vi "OldClient.vi"() -> ()   [LabVIEW 2025]
uses:
  common/CommonClientNetworkInterfaceGlobalVariables.vi
  ClientGlobalVariables.vi
  ClientNetworkInterfaceGlobalVariables.vi
panel:
  out "ACTION":T1
  in  "Array":string[][](array[string])
  in  "Team":u8=1 max=15 step=1
  in  "Tab Control":enum32{"start", "PreGame", "InGame"}(tab)
  in  "ServerAddress":string
  in  "exit":bool
  in  "play":bool
  out "Status":string
  in  "PlayerName":string
  in  "leave game":bool
  in  "PreGame menu":enum32{"Team", "Options"}(tab)
  in  "spectator":bool caption="Blank Button"
  in  "team5":bool caption="Blank Button"
  in  "team4":bool caption="Blank Button"
  in  "team3":bool caption="Blank Button"
  in  "team2":bool caption="Blank Button"
  in  "team1":bool caption="Blank Button"
  out "Lobby Player List":T2(array[cluster])
  in  "Speed":i32(slide) caption="Slide" scale=1.0..4.0
  in  "Map Width":i32(slide) caption="Slide" scale=10.0..40.0
  in  "Map Height":i32(slide) caption="Slide" scale=10.0..40.0
  in  "City Density":i32(slide) caption="Slide" scale=20.0..80.0
  in  "Mountain Density":i32(slide) caption="Slide" scale=20.0..80.0
  out "Status 2":string
  in  "Ready":bool
  in  "back_to _lobby":bool
  out "Turns":string
  in  "play 2":bool
  out "Game Field":picture
  out "In-game Player List":string[][](table) caption="Table Control"
  # "generals.io"
  # "generals.io"
  # "Protect your general. Capture enemy generals."
  # "Player Name"
  # "Server Address"
  # "Status"
  # "Status"
  # "select your team"
  # "Team"
  # "Turn"
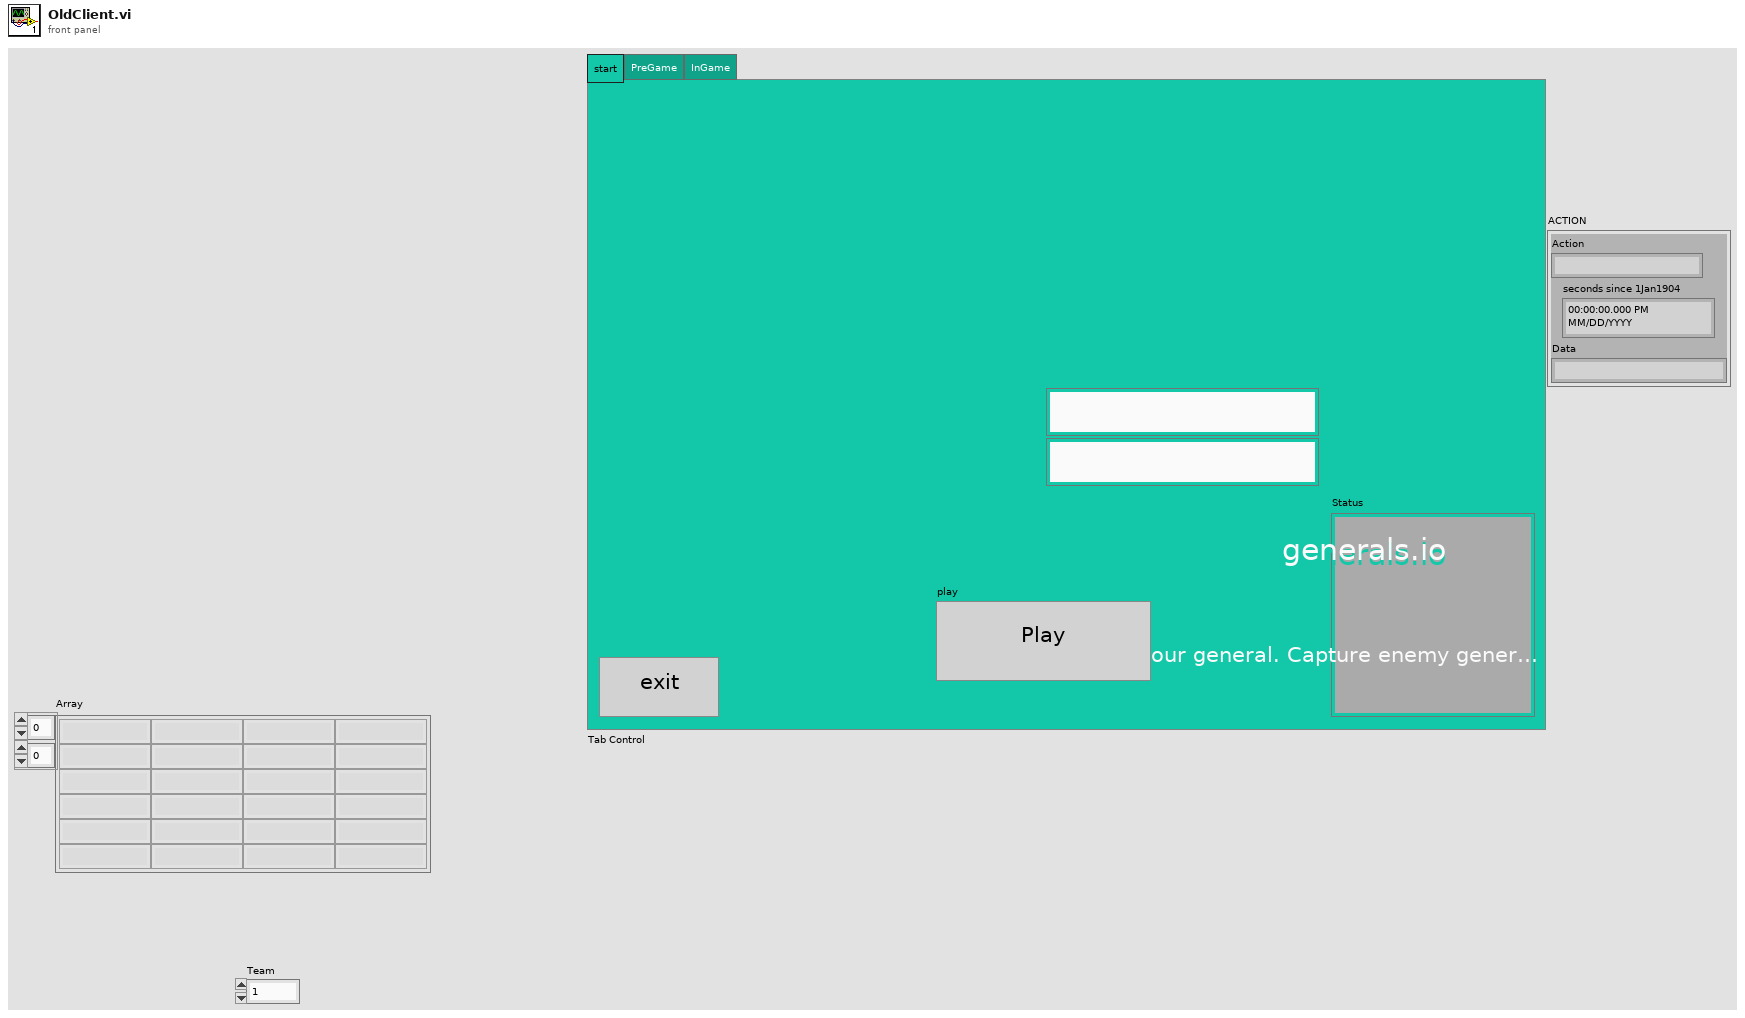
[diagram p1: front panel]
types:
  T1 = cluster{"Action":string, "seconds since 1Jan1904":timestamp, "Data":string}
  T2 = cluster{"Color":u32, "Host":bool, "Name":string, "Team":u8, "Ready":bool}[]
  T3 = cluster{"seconds since 1Jan1904":timestamp, "Data":string}
  T4 = enum16{"Wait Send Queue Ready", "Wait Receive Queue Ready", "Poll Read Queue", "Process Data"}
  T5 = typedef "LVPoint32TypeDef.ctl" = cluster{"Horizontal":i32, "Vertical":i32}
  T6 = cluster{"Round":u32, "FieldArray":cluster{"Troops":u32, "Owner":i32, "Mountain":bool, "City":bool, "General":bool, "Fog":bool}[][]}
  T7 = cluster{"Troops":u32, "Owner":i32, "Mountain":bool, "City":bool, "General":bool, "Fog":bool}[][]
  T8 = map{u32, cluster{"Name":string, "Team":u8, "Ready":bool, "Host":bool, "Alive":bool, "Color":u32, "Lands":set{cluster{"Row":u32, "Column":u32}}, "Army":u32}}
  T9 = cluster{"Color":u32, "Host":bool, "Name":string, "Team":u8, "Ready":bool}
  T10 = cluster{"Lands":set{cluster{"Row":u32, "Column":u32}}}[]
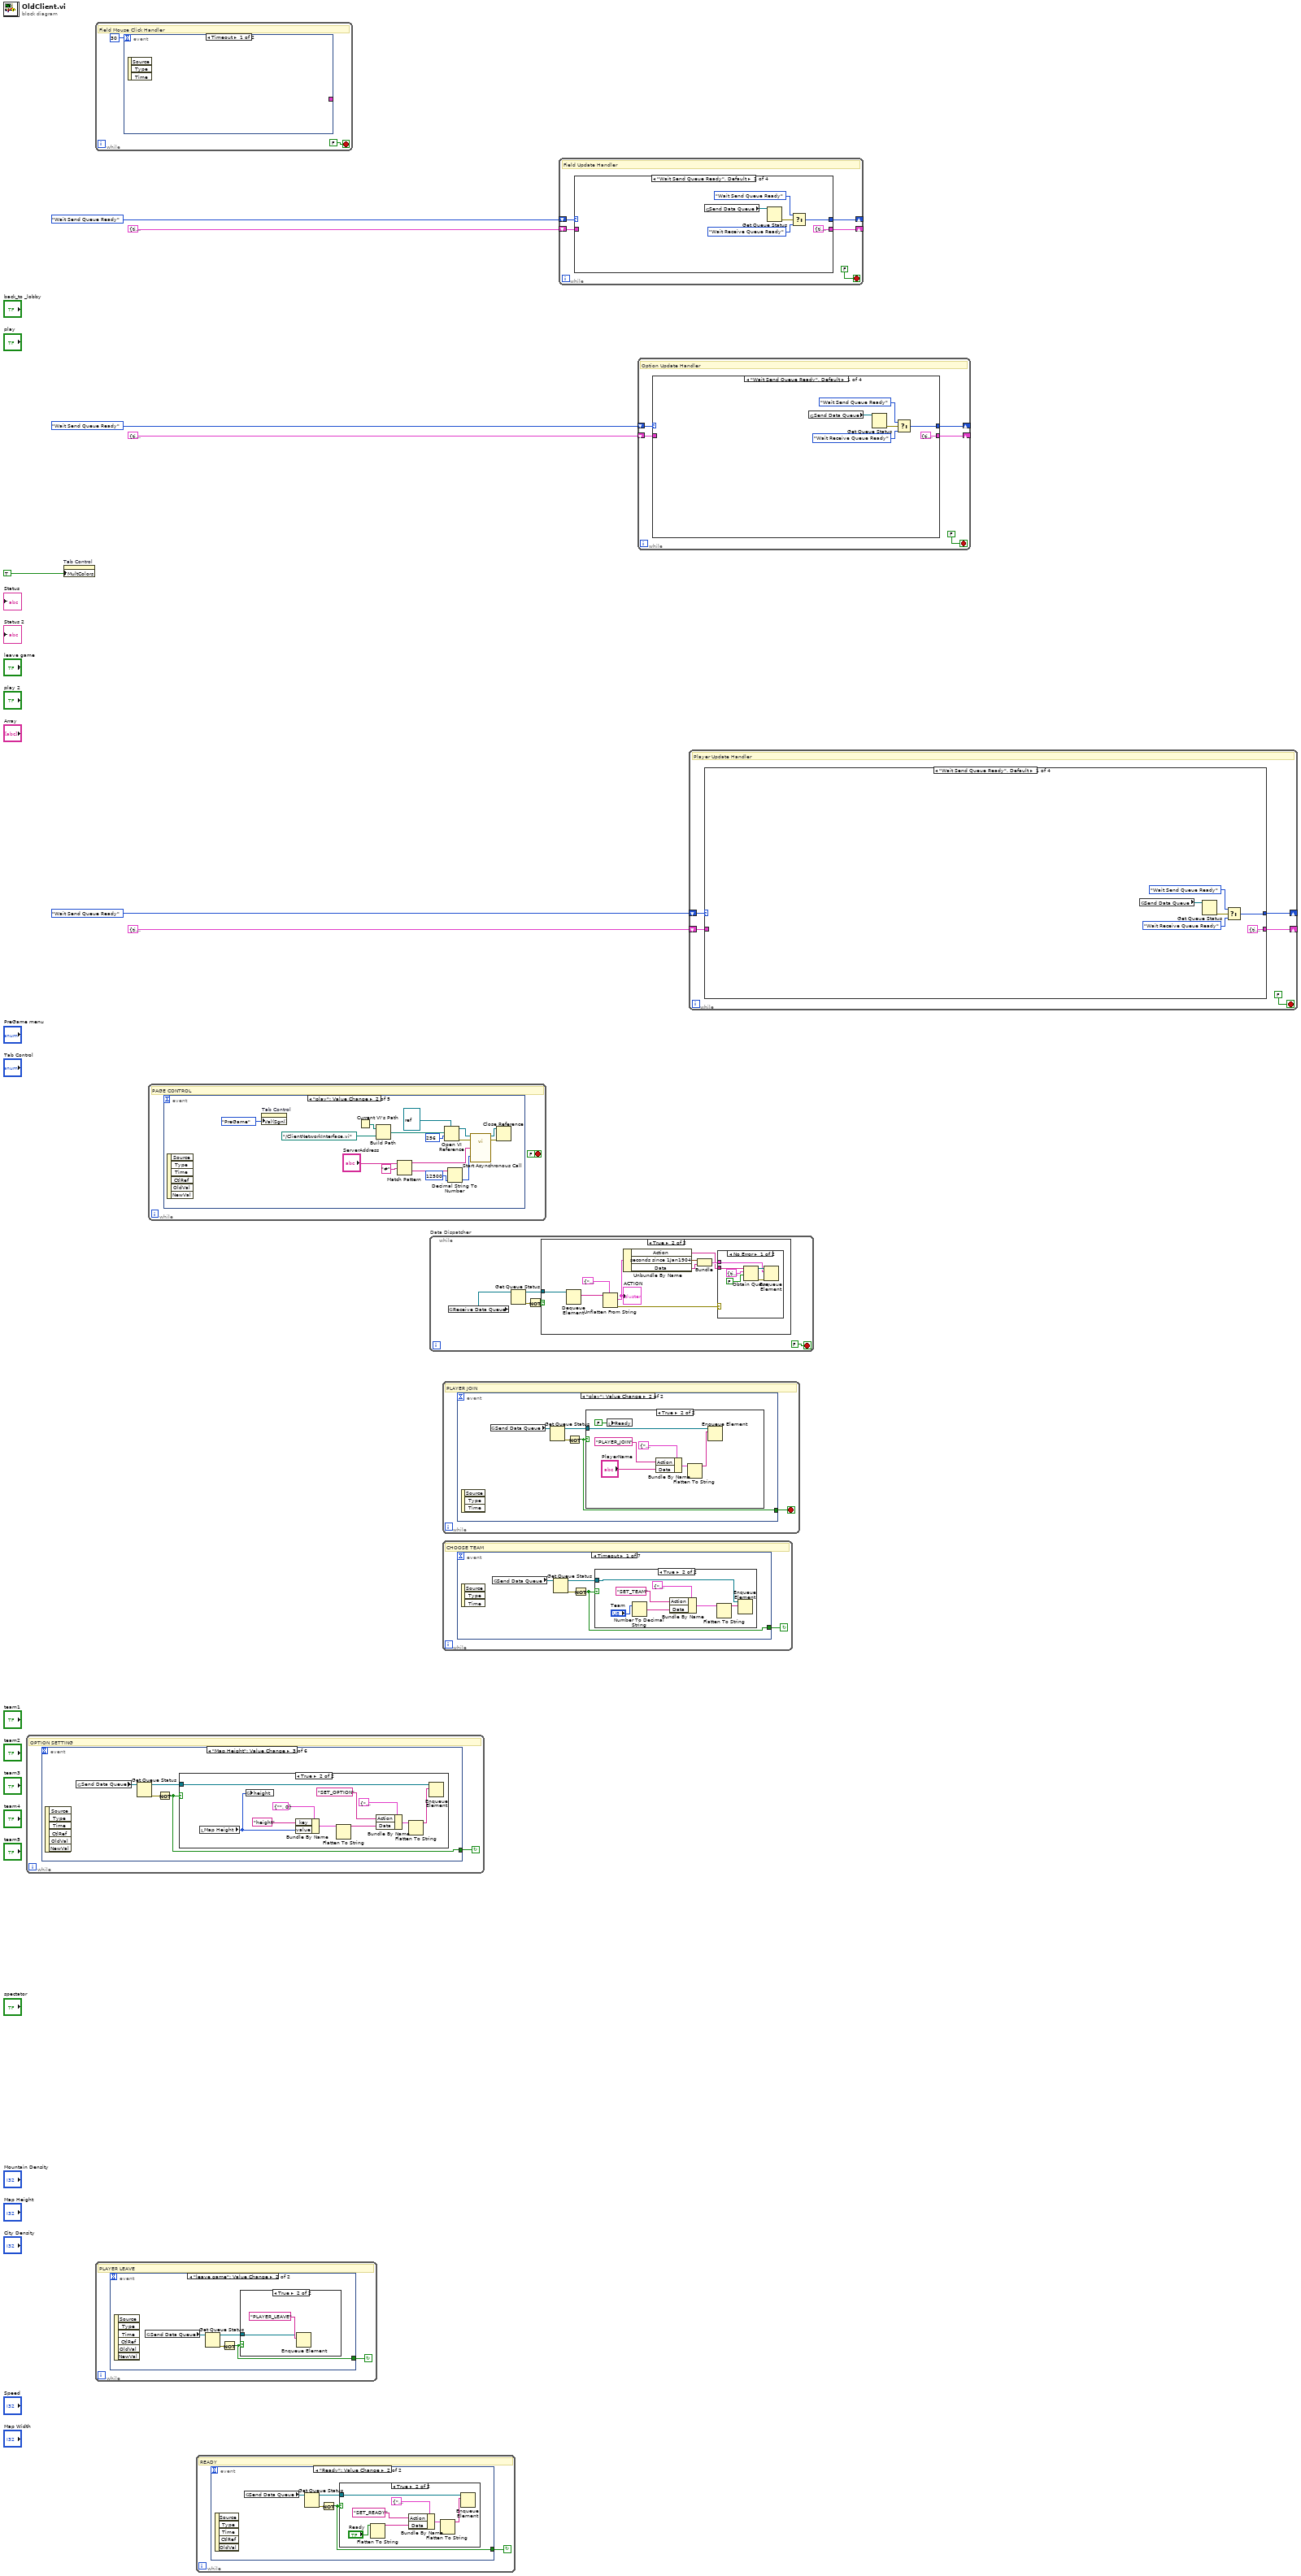
[diagram p0: block diagram]
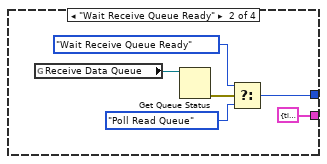
[diagram p2: hidden frame]
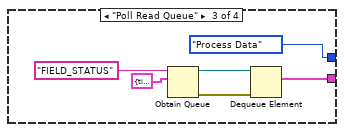
[diagram p3: hidden frame]
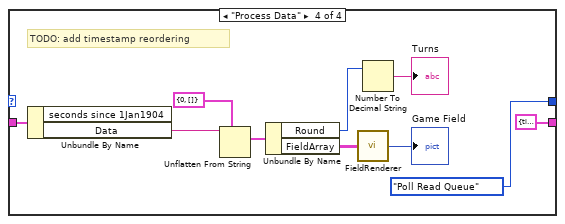
[diagram p4: hidden frame]
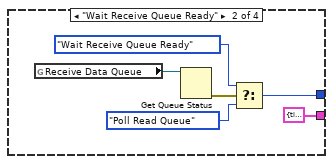
[diagram p5: hidden frame]
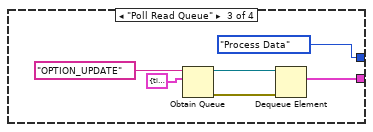
[diagram p6: hidden frame]
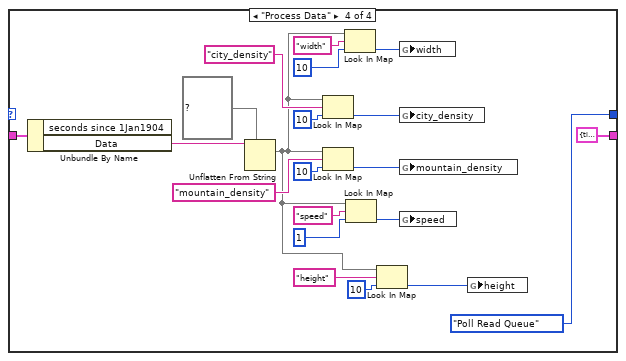
[diagram p7: hidden frame]
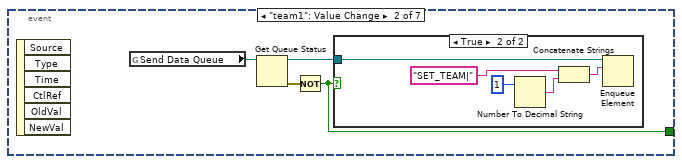
[diagram p9: hidden frame]
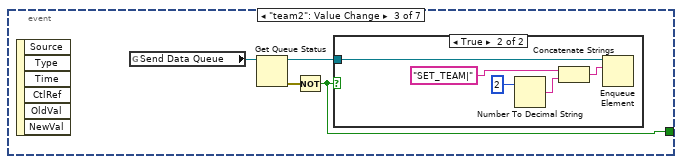
[diagram p11: hidden frame]
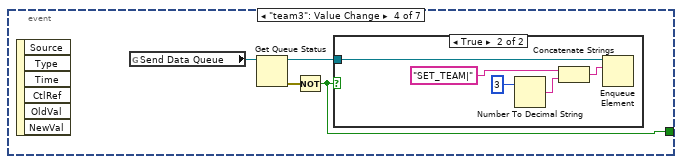
[diagram p13: hidden frame]
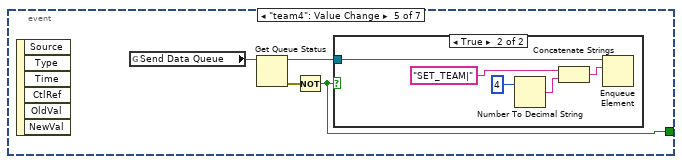
[diagram p15: hidden frame]
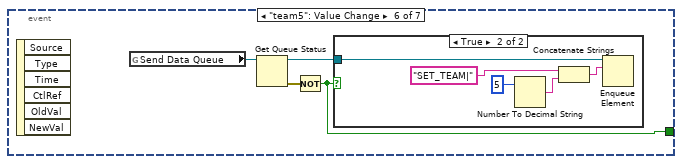
[diagram p17: hidden frame]
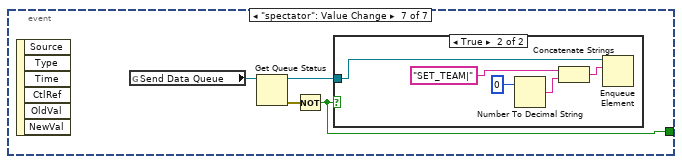
[diagram p19: hidden frame]
diagram:
  n1 = while {
    stop <- w8 continue-if-true
    # "OPTION SETTING"
    n2 = event shown="[2] \"Map Height\": Value Change" {
      selector: _ -> [_ _ _ _ _ _]
      dyn-events: _ -> [_ _ _ _ _ _]
      timeout: _ -> [_ _ _ _ _ _]
      tunnel: [_ w9 w24 w37 w51 w66] -> w8
      event Timeout {
        n3 = event-data() -> ()  [unwired: 1 in, 3 out]
      }
      event "Map Width": Value Change {
        n4 = event-data() -> ()  [unwired: 1 in, 6 out]
        n5 = global read "CommonClientNetworkInterfaceGlobalVariables.vi" "Send Data Queue"() -> (w11:refnum<queue>)
        n6 = Get Queue Status(queue=w11) -> (queue out=w10:refnum<queue>, error out=w12:errorcluster)  [unwired: 2 in, 6 out]
        n7 = Not(x=w12) -> (.not. x?=w9:bool)
        n8 = case shown="True" w9 {
          tunnel: w10 -> [_ w22]
          frame False {
          }
          frame True {
            n9 = local read "Map Width"() -> (w19:i32)
            n10 = global write "ClientGlobalVariables.vi" "width"(w19) -> ()
            n11 = Bundle By Name(cluster=cluster{"key":string, "value":u32} {"key"="", "value"=0}, "key"="width" ("Option"), "value"=w19) -> (w15:cluster{"key":string, "value":u32})
            n12 = Flatten To String(anything=w15) -> (data string=w16:string)  [unwired: 3 in, 2 out]
            n13 = Bundle By Name(cluster=cluster{"Action":string, "Data":string} {"Action"="", "Data"=""} ("CommandCluster"), "Action"="SET_OPTION" ("string"), "Data"=w16) -> (w13:cluster{"Action":string, "Data":string})
            n14 = Flatten To String(anything=w13) -> (data string=w14:string)  [unwired: 3 in, 2 out]
            n15 = Enqueue Element(queue=w22, element=w14) -> ()  [unwired: 2 in, 3 out]
          }
        }
      }
      event "Map Height": Value Change {
        n16 = event-data() -> ()  [unwired: 1 in, 6 out]
        n17 = global read "CommonClientNetworkInterfaceGlobalVariables.vi" "Send Data Queue"() -> (w25:refnum<queue>)
        n18 = Get Queue Status(queue=w25) -> (queue out=w23:refnum<queue>, error out=w26:errorcluster)  [unwired: 2 in, 6 out]
        n19 = Not(x=w26) -> (.not. x?=w24:bool)
        n20 = case shown="True" w24 {
          tunnel: w23 -> [_ w28]
          frame False {
          }
          frame True {
            n21 = local read "Map Height"() -> (w27:i32)
            n22 = global write "ClientGlobalVariables.vi" "height"(w27) -> ()
            n23 = Bundle By Name(cluster=cluster{"key":string, "value":u32} {"key"="", "value"=0}, "key"="height" ("Option"), "value"=w27) -> (w31:cluster{"key":string, "value":u32})
            n24 = Flatten To String(anything=w31) -> (data string=w32:string)  [unwired: 3 in, 2 out]
            n25 = Bundle By Name(cluster=cluster{"Action":string, "Data":string} {"Action"="", "Data"=""} ("CommandCluster"), "Action"="SET_OPTION" ("string"), "Data"=w32) -> (w29:cluster{"Action":string, "Data":string})
            n26 = Flatten To String(anything=w29) -> (data string=w30:string)  [unwired: 3 in, 2 out]
            n27 = Enqueue Element(queue=w28, element=w30) -> ()  [unwired: 2 in, 3 out]
          }
        }
      }
      event "Speed": Value Change {
        n28 = event-data() -> ()  [unwired: 1 in, 6 out]
        n29 = global read "CommonClientNetworkInterfaceGlobalVariables.vi" "Send Data Queue"() -> (w39:refnum<queue>)
        n30 = Get Queue Status(queue=w39) -> (queue out=w38:refnum<queue>, error out=w40:errorcluster)  [unwired: 2 in, 6 out]
        n31 = Not(x=w40) -> (.not. x?=w37:bool)
        n32 = case shown="True" w37 {
          tunnel: w38 -> [_ w41]
          frame False {
          }
          frame True {
            n33 = local read "Speed"() -> (w42:i32)
            n34 = global write "ClientGlobalVariables.vi" "speed"(w42) -> ()
            n35 = Bundle By Name(cluster=cluster{"key":string, "value":u32} {"key"="", "value"=0}, "key"="speed" ("Option"), "value"=w42) -> (w45:cluster{"key":string, "value":u32})
            n36 = Flatten To String(anything=w45) -> (data string=w46:string)  [unwired: 3 in, 2 out]
            n37 = Bundle By Name(cluster=cluster{"Action":string, "Data":string} {"Action"="", "Data"=""} ("CommandCluster"), "Action"="SET_OPTION" ("string"), "Data"=w46) -> (w43:cluster{"Action":string, "Data":string})
            n38 = Flatten To String(anything=w43) -> (data string=w44:string)  [unwired: 3 in, 2 out]
            n39 = Enqueue Element(queue=w41, element=w44) -> ()  [unwired: 2 in, 3 out]
          }
        }
      }
      event "Mountain Density": Value Change {
        n40 = event-data() -> ()  [unwired: 1 in, 6 out]
        n41 = global read "CommonClientNetworkInterfaceGlobalVariables.vi" "Send Data Queue"() -> (w53:refnum<queue>)
        n42 = Get Queue Status(queue=w53) -> (queue out=w52:refnum<queue>, error out=w54:errorcluster)  [unwired: 2 in, 6 out]
        n43 = Not(x=w54) -> (.not. x?=w51:bool)
        n44 = case shown="True" w51 {
          tunnel: w52 -> [_ w56]
          frame False {
          }
          frame True {
            n45 = local read "Mountain Density"() -> (w55:i32)
            n46 = global write "ClientGlobalVariables.vi" "mountain_density"(w55) -> ()
            n47 = Bundle By Name(cluster=cluster{"key":string, "value":u32} {"key"="", "value"=0}, "key"="mountain_density" ("Option"), "value"=w55) -> (w59:cluster{"key":string, "value":u32})
            n48 = Flatten To String(anything=w59) -> (data string=w60:string)  [unwired: 3 in, 2 out]
            n49 = Bundle By Name(cluster=cluster{"Action":string, "Data":string} {"Action"="", "Data"=""} ("CommandCluster"), "Action"="SET_OPTION" ("string"), "Data"=w60) -> (w57:cluster{"Action":string, "Data":string})
            n50 = Flatten To String(anything=w57) -> (data string=w58:string)  [unwired: 3 in, 2 out]
            n51 = Enqueue Element(queue=w56, element=w58) -> ()  [unwired: 2 in, 3 out]
          }
        }
      }
      event "City Density": Value Change {
        n52 = event-data() -> ()  [unwired: 1 in, 6 out]
        n53 = global read "CommonClientNetworkInterfaceGlobalVariables.vi" "Send Data Queue"() -> (w67:refnum<queue>)
        n54 = Get Queue Status(queue=w67) -> (queue out=w65:refnum<queue>, error out=w68:errorcluster)  [unwired: 2 in, 6 out]
        n55 = Not(x=w68) -> (.not. x?=w66:bool)
        n56 = case shown="True" w66 {
          tunnel: w65 -> [_ w69]
          frame False {
          }
          frame True {
            n57 = local read "City Density"() -> (w70:i32)
            n58 = global write "ClientGlobalVariables.vi" "city_density"(w70) -> ()
            n59 = Bundle By Name(cluster=cluster{"key":string, "value":u32} {"key"="", "value"=0}, "key"="city_density" ("Option"), "value"=w70) -> (w73:cluster{"key":string, "value":u32})
            n60 = Flatten To String(anything=w73) -> (data string=w74:string)  [unwired: 3 in, 2 out]
            n61 = Bundle By Name(cluster=cluster{"Action":string, "Data":string} {"Action"="", "Data"=""} ("CommandCluster"), "Action"="SET_OPTION" ("string"), "Data"=w74) -> (w71:cluster{"Action":string, "Data":string})
            n62 = Flatten To String(anything=w71) -> (data string=w72:string)  [unwired: 3 in, 2 out]
            n63 = Enqueue Element(queue=w69, element=w72) -> ()  [unwired: 2 in, 3 out]
          }
        }
      }
    }
  }
  n64 = property on="Tab Control" class="TabCtl (strict)"("MultColors"=TRUE ("Allow Multiple Colors")) -> ()  [unwired: 2 in, 2 out]
  n65 = while {
    stop <- FALSE stop-if-true
    # "Field Mouse Click Handler"
    n66 = event shown="[0] Timeout" {
      selector: _ -> [_ _]
      dyn-events: _ -> [_ _]
      timeout: 30 -> [_ _]
      tunnel: [_ w94] -> _
      event Timeout {
        n67 = event-data() -> ()  [unwired: 1 in, 3 out]
      }
      event "Game Field": Mouse Down {
        # "col"
        # "row"
        n68 = event-data() -> ("Coords"=w96:T5)  [unwired: 1 in, 7 out]
        n69 = Unbundle By Name(w96) -> ("Horizontal"=w93:i32, "Vertical"=w92:i32)
        n70 = global read "ClientGlobalVariables.vi" "FieldLength"() -> (w83:i32)
        n71 = global read "ClientGlobalVariables.vi" "height"() -> (w84:i32)
        n72 = global read "ClientGlobalVariables.vi" "width"() -> (w85:i32)
        n73 = Quotient & Remainder(x=w83, y=w85) -> (floor(x/y)=w82:i32)  [unwired: 1 out]
        n74 = Quotient & Remainder(x=w83, y=w84) -> (floor(x/y)=w81:i32)  [unwired: 1 out]
        n75 = Quotient & Remainder(x=w93, y=w82) -> (floor(x/y)=w90:i32)  [unwired: 1 out]
        n76 = Quotient & Remainder(x=w92, y=w81) -> (floor(x/y)=w88:i32)  [unwired: 1 out]
        n77 = Subtract(x=w88, y=4) -> (x-y=w87:i32)
        n78 = Subtract(x=w90, y=13) -> (x-y=w91:i32)
        n79 = Bundle(w91, w87, TRUE) -> (w94:cluster{i32, i32, bool})  [unwired: 1 in]
      }
    }
  }
  n80 = while {
    stop <- w97 continue-if-true
    # "PLAYER LEAVE"
    n81 = event shown="[1] \"leave game\": Value Change" {
      selector: _ -> [_ _]
      dyn-events: _ -> [_ _]
      timeout: _ -> [_ _]
      tunnel: [_ w99] -> w97
      event Timeout {
        n82 = event-data() -> ()  [unwired: 1 in, 3 out]
      }
      event "leave game": Value Change {
        n83 = event-data() -> ()  [unwired: 1 in, 6 out]
        n84 = global read "CommonClientNetworkInterfaceGlobalVariables.vi" "Send Data Queue"() -> (w100:refnum<queue>)
        n85 = Get Queue Status(queue=w100) -> (queue out=w98:refnum<queue>, error out=w101:errorcluster)  [unwired: 2 in, 6 out]
        n86 = Not(x=w101) -> (.not. x?=w99:bool)
        n87 = case shown="True" w99 {
          tunnel: w98 -> [_ w102]
          frame False {
          }
          frame True {
            n88 = Enqueue Element(queue=w102, element="PLAYER_LEAVE" ("string")) -> ()  [unwired: 2 in, 3 out]
          }
        }
      }
    }
  }
  n89 = while {
    stop <- FALSE stop-if-true
    # "PAGE CONTROL"
    n90 = event shown="[1] \"play\": Value Change" {
      selector: _ -> [_ _ _ _ _]
      dyn-events: _ -> [_ _ _ _ _]
      timeout: _ -> [_ _ _ _ _]
      event Timeout {
        n91 = event-data() -> ()  [unwired: 1 in, 3 out]
      }
      event "play": Value Change {
        n92 = event-data() -> ()  [unwired: 1 in, 6 out]
        n93 = property on="Tab Control" class="TabCtl (strict)"("Val(Sgnl)"=enum32{"start", "PreGame", "InGame"}."PreGame" ("Value (Signaling)")) -> ()  [unwired: 2 in, 2 out]
        n94 = Current VI's Path() -> (path=w115:path)
        n95 = Build Path(base path=w115, name or relative path=path "../ClientNetworkInterface.vi" ("vi path")) -> (appended path=w113:path)
        n96 = Match Pattern(string="ServerAddress", regular expression="#") -> (before substring=w106:string, after substring=w119:string)  [unwired: 1 in, 2 out]
        n97 = Open VI Reference(type specifier VI Refnum (for type only)=refnum<vi> refnum ("VI Refnum"), vi path=w113, options=256) -> (vi reference=w107:refnum<vi>, error out=w111:errorcluster)  [unwired: 3 in]
        n98 = Decimal String To Number(string=w119, default (0L)=u16 12500 ("Server Port")) -> (number=w105:u16)  [unwired: 1 in, 1 out]
        n99 = call-by-ref "Start Asynchronous Call"(reference=w107, error in=w111, "Server Port"=w105, "Server Address"=w106) -> (reference out=w110:refnum<vi>, error out=w109:errorcluster)
        n100 = Close Reference(reference=w110, error in (no error)=w109) -> ()  [unwired: 1 out]
      }
      event "leave game": Value Change {
        n101 = event-data() -> ()  [unwired: 1 in, 6 out]
        n102 = property on="Tab Control" class="TabCtl (strict)"("Val(Sgnl)"=enum32{"start", "PreGame", "InGame"}."start" ("Value (Signaling)")) -> ()  [unwired: 2 in, 2 out]
      }
      event "back_to _lobby": Value Change {
        n103 = event-data() -> ()  [unwired: 1 in, 6 out]
        n104 = local read "Speed"() -> (w126:i32)
        n105 = local read "Map Height"() -> (w125:i32)
        n106 = local read "City Density"() -> (w123:i32)
        n107 = local read "Map Width"() -> (w124:i32)
        n108 = global write "ClientGlobalVariables.vi" "FieldLength"(600 ("FieldLength")) -> ()
        n109 = global write "ClientGlobalVariables.vi" "speed"(w126) -> ()
        n110 = local read "Mountain Density"() -> (w127:i32)
        n111 = global write "ClientGlobalVariables.vi" "city_density"(w123) -> ()
        n112 = global write "ClientGlobalVariables.vi" "height"(w125) -> ()
        n113 = global write "ClientGlobalVariables.vi" "width"(w124) -> ()
        n114 = property on="Tab Control" class="TabCtl (strict)"("Val(Sgnl)"=enum32{"start", "PreGame", "InGame"}."PreGame" ("Value (Signaling)")) -> ()  [unwired: 2 in, 2 out]
        n115 = global write "ClientGlobalVariables.vi" "mountain_density"(w127) -> ()
      }
      event "exit": Value Change {
        n116 = event-data() -> ()  [unwired: 1 in, 6 out]
        n117 = Quit LabVIEW(quit? (T)="exit") -> ()
      }
    }
  }
  n118 = while {
    stop <- w130 continue-if-true
    # "READY"
    n119 = event shown="[1] \"Ready\": Value Change" {
      selector: _ -> [_ _]
      dyn-events: _ -> [_ _]
      timeout: _ -> [_ _]
      tunnel: [_ w131] -> w130
      event Timeout {
        n120 = event-data() -> ()  [unwired: 1 in, 3 out]
      }
      event "Ready": Value Change {
        n121 = event-data() -> ()  [unwired: 1 in, 5 out]
        n122 = global read "CommonClientNetworkInterfaceGlobalVariables.vi" "Send Data Queue"() -> (w134:refnum<queue>)
        n123 = Get Queue Status(queue=w134) -> (queue out=w133:refnum<queue>, error out=w132:errorcluster)  [unwired: 2 in, 6 out]
        n124 = Not(x=w132) -> (.not. x?=w131:bool)
        n125 = case shown="True" w131 {
          tunnel: w133 -> [_ w135]
          frame False {
          }
          frame True {
            n126 = Flatten To String(anything="Ready") -> (data string=w139:string)  [unwired: 3 in, 2 out]
            n127 = Bundle By Name(cluster=cluster{"Action":string, "Data":string} {"Action"="", "Data"=""} ("CommandCluster"), "Action"="SET_READY" ("string"), "Data"=w139) -> (w137:cluster{"Action":string, "Data":string})
            n128 = Flatten To String(anything=w137) -> (data string=w138:string)  [unwired: 3 in, 2 out]
            n129 = Enqueue Element(queue=w135, element=w138) -> ()  [unwired: 2 in, 3 out]
          }
        }
      }
    }
  }
  n130 = while "Data Dispatcher" {
    stop <- FALSE stop-if-true
    n131 = global read "ClientNetworkInterfaceGlobalVariables.vi" "Receive Data Queue"() -> (w142:refnum<queue>)
    n132 = Get Queue Status(queue=w142) -> (queue out=w143:refnum<queue>, error out=w145:errorcluster)  [unwired: 2 in, 6 out]
    n133 = Not(x=w145) -> (.not. x?=w144:bool)
    n134 = case shown="True" w144 {
      tunnel: w143 -> [_ w155]
      frame False {
      }
      frame True {
        n135 = Dequeue Element(queue=w155) -> (element=w154:string)  [unwired: 2 in, 3 out]
        n136 = Unflatten From String(type=T1 {"Action"="", "seconds since 1Jan1904"=timestamp(0 s since 1904-01-01), "Data"=""} ("CommandCluster"), binary string=w154) -> (value=w147:T1, error out=w148:errorcluster)  [unwired: 3 in, 1 out]
        "ACTION" <- w147
        n137 = Unbundle By Name(w147) -> ("Action"=w149:string, "seconds since 1Jan1904"=w152:timestamp, "Data"=w151:string)
        n138 = Bundle("seconds since 1Jan1904"=w152, "Data"=w151) -> (w150:T3)  [unwired: 1 in]
        n139 = case shown="No Error" w148 {
          tunnel: w150 -> [w158 _]
          tunnel: w149 -> [w157 _]
          frame No Error {
            n140 = Obtain Queue(name (unnamed)=w157, element data type=T3 {"seconds since 1Jan1904"=timestamp(0 s since 1904-01-01), "Data"=""} ("ActionDataCluster"), create if not found? (T)=FALSE) -> (queue out=w160:refnum<queue>, error out=w159:errorcluster)  [unwired: 2 in, 1 out]
            n141 = Enqueue Element(queue=w160, element=w158, error in (no error)=w159) -> ()  [unwired: 1 in, 3 out]
          }
          frame Error {
          }
        }
      }
    }
  }
  n142 = while {
    stop <- w162 stop-if-true
    # "PLAYER JOIN"
    n143 = event shown="[1] \"play\": Value Change" {
      selector: _ -> [_ _]
      dyn-events: _ -> [_ _]
      timeout: _ -> [_ _]
      tunnel: [_ w164] -> w162
      event Timeout {
        n144 = event-data() -> ()  [unwired: 1 in, 3 out]
      }
      event "play": Value Change {
        n145 = event-data() -> ()  [unwired: 1 in, 3 out]
        n146 = global read "ClientNetworkInterfaceGlobalVariables.vi" "Send Data Queue"() -> (w163:refnum<queue>)
        n147 = Get Queue Status(queue=w163) -> (queue out=w165:refnum<queue>, error out=w166:errorcluster)  [unwired: 2 in, 6 out]
        n148 = Not(x=w166) -> (.not. x?=w164:bool)
        n149 = case shown="True" w164 {
          tunnel: w165 -> [_ w173]
          frame False {
          }
          frame True {
            n150 = local write "Ready"(FALSE ("Ready")) -> ()
            n151 = Bundle By Name(cluster=cluster{"Action":string, "Data":string} {"Action"="", "Data"=""} ("CommandCluster"), "Action"="PLAYER_JOIN" ("string"), "Data"="PlayerName") -> (w168:cluster{"Action":string, "Data":string})
            n152 = Flatten To String(anything=w168) -> (data string=w167:string)  [unwired: 3 in, 2 out]
            n153 = Enqueue Element(queue=w173, element=w167) -> ()  [unwired: 2 in, 3 out]
          }
        }
      }
    }
  }
  n154 = while {
    stop <- w174 continue-if-true
    # "CHOOSE TEAM"
    n155 = event shown="[0] Timeout" {
      selector: _ -> [_ _ _ _ _ _ _]
      dyn-events: _ -> [_ _ _ _ _ _ _]
      timeout: _ -> [_ _ _ _ _ _ _]
      tunnel: [w176 w187 w196 w205 w214 w223 w232] -> w174
      event Timeout {
        n156 = event-data() -> ()  [unwired: 1 in, 3 out]
        n157 = global read "CommonClientNetworkInterfaceGlobalVariables.vi" "Send Data Queue"() -> (w178:refnum<queue>)
        n158 = Get Queue Status(queue=w178) -> (queue out=w175:refnum<queue>, error out=w177:errorcluster)  [unwired: 2 in, 6 out]
        n159 = Not(x=w177) -> (.not. x?=w176:bool)
        n160 = case shown="True" w176 {
          tunnel: w175 -> [_ w185]
          frame False {
          }
          frame True {
            n161 = Number To Decimal String(number="Team") -> (decimal integer string=w180:string)  [unwired: 1 in]
            n162 = Bundle By Name(cluster=cluster{"Action":string, "Data":string} {"Action"="", "Data"=""} ("CommandCluster"), "Action"="SET_TEAM" ("string"), "Data"=w180) -> (w181:cluster{"Action":string, "Data":string})
            n163 = Flatten To String(anything=w181) -> (data string=w179:string)  [unwired: 3 in, 2 out]
            n164 = Enqueue Element(queue=w185, element=w179) -> ()  [unwired: 2 in, 3 out]
          }
        }
      }
      event "team1": Value Change {
        n165 = event-data() -> ()  [unwired: 1 in, 6 out]
        n166 = global read "CommonClientNetworkInterfaceGlobalVariables.vi" "Send Data Queue"() -> (w189:refnum<queue>)
        n167 = Get Queue Status(queue=w189) -> (queue out=w186:refnum<queue>, error out=w188:errorcluster)  [unwired: 2 in, 6 out]
        n168 = Not(x=w188) -> (.not. x?=w187:bool)
        n169 = case shown="True" w187 {
          tunnel: w186 -> [_ w191]
          frame False {
          }
          frame True {
            n170 = Number To Decimal String(number=1) -> (decimal integer string=w192:string)  [unwired: 1 in]
            n171 = Concatenate Strings("SET_TEAM|" ("string"), w192) -> (w193:string)
            n172 = Enqueue Element(queue=w191, element=w193) -> ()  [unwired: 2 in, 3 out]
          }
        }
      }
      event "team2": Value Change {
        n173 = event-data() -> ()  [unwired: 1 in, 6 out]
        n174 = global read "CommonClientNetworkInterfaceGlobalVariables.vi" "Send Data Queue"() -> (w198:refnum<queue>)
        n175 = Get Queue Status(queue=w198) -> (queue out=w195:refnum<queue>, error out=w197:errorcluster)  [unwired: 2 in, 6 out]
        n176 = Not(x=w197) -> (.not. x?=w196:bool)
        n177 = case shown="True" w196 {
          tunnel: w195 -> [_ w200]
          frame False {
          }
          frame True {
            n178 = Number To Decimal String(number=2) -> (decimal integer string=w201:string)  [unwired: 1 in]
            n179 = Concatenate Strings("SET_TEAM|" ("string"), w201) -> (w202:string)
            n180 = Enqueue Element(queue=w200, element=w202) -> ()  [unwired: 2 in, 3 out]
          }
        }
      }
      event "team3": Value Change {
        n181 = event-data() -> ()  [unwired: 1 in, 6 out]
        n182 = global read "CommonClientNetworkInterfaceGlobalVariables.vi" "Send Data Queue"() -> (w207:refnum<queue>)
        n183 = Get Queue Status(queue=w207) -> (queue out=w204:refnum<queue>, error out=w206:errorcluster)  [unwired: 2 in, 6 out]
        n184 = Not(x=w206) -> (.not. x?=w205:bool)
        n185 = case shown="True" w205 {
          tunnel: w204 -> [_ w209]
          frame False {
          }
          frame True {
            n186 = Number To Decimal String(number=3) -> (decimal integer string=w210:string)  [unwired: 1 in]
            n187 = Concatenate Strings("SET_TEAM|" ("string"), w210) -> (w211:string)
            n188 = Enqueue Element(queue=w209, element=w211) -> ()  [unwired: 2 in, 3 out]
          }
        }
      }
      event "team4": Value Change {
        n189 = event-data() -> ()  [unwired: 1 in, 6 out]
        n190 = global read "CommonClientNetworkInterfaceGlobalVariables.vi" "Send Data Queue"() -> (w216:refnum<queue>)
        n191 = Get Queue Status(queue=w216) -> (queue out=w213:refnum<queue>, error out=w215:errorcluster)  [unwired: 2 in, 6 out]
        n192 = Not(x=w215) -> (.not. x?=w214:bool)
        n193 = case shown="True" w214 {
          tunnel: w213 -> [_ w218]
          frame False {
          }
          frame True {
            n194 = Number To Decimal String(number=4) -> (decimal integer string=w219:string)  [unwired: 1 in]
            n195 = Concatenate Strings("SET_TEAM|" ("string"), w219) -> (w220:string)
            n196 = Enqueue Element(queue=w218, element=w220) -> ()  [unwired: 2 in, 3 out]
          }
        }
      }
      event "team5": Value Change {
        n197 = event-data() -> ()  [unwired: 1 in, 6 out]
        n198 = global read "CommonClientNetworkInterfaceGlobalVariables.vi" "Send Data Queue"() -> (w225:refnum<queue>)
        n199 = Get Queue Status(queue=w225) -> (queue out=w222:refnum<queue>, error out=w224:errorcluster)  [unwired: 2 in, 6 out]
        n200 = Not(x=w224) -> (.not. x?=w223:bool)
        n201 = case shown="True" w223 {
          tunnel: w222 -> [_ w227]
          frame False {
          }
          frame True {
            n202 = Number To Decimal String(number=5) -> (decimal integer string=w228:string)  [unwired: 1 in]
            n203 = Concatenate Strings("SET_TEAM|" ("string"), w228) -> (w229:string)
            n204 = Enqueue Element(queue=w227, element=w229) -> ()  [unwired: 2 in, 3 out]
          }
        }
      }
      event "spectator": Value Change {
        n205 = event-data() -> ()  [unwired: 1 in, 6 out]
        n206 = global read "CommonClientNetworkInterfaceGlobalVariables.vi" "Send Data Queue"() -> (w234:refnum<queue>)
        n207 = Get Queue Status(queue=w234) -> (queue out=w231:refnum<queue>, error out=w233:errorcluster)  [unwired: 2 in, 6 out]
        n208 = Not(x=w233) -> (.not. x?=w232:bool)
        n209 = case shown="True" w232 {
          tunnel: w231 -> [_ w236]
          frame False {
          }
          frame True {
            n210 = Number To Decimal String(number=0) -> (decimal integer string=w237:string)  [unwired: 1 in]
            n211 = Concatenate Strings("SET_TEAM|" ("string"), w237) -> (w238:string)
            n212 = Enqueue Element(queue=w236, element=w238) -> ()  [unwired: 2 in, 3 out]
          }
        }
      }
    }
  }
  n213 = while {
    shift-right: [w243] -> _
    shift-left: T4."Wait Send Queue Ready" -> [w242]
    shift-right: [w241] -> _
    shift-left: T3 {"seconds since 1Jan1904"=timestamp(0 s since 1904-01-01), "Data"=""} ("ActionDataCluster") -> [w240]
    stop <- FALSE stop-if-true
    # "Field Update Handler"
    n214 = case shown="\"Wait Send Queue Ready\", Default" w242 {
      tunnel: [w249 w253 T4."Process Data" T4."Poll Read Queue"] -> w243
      tunnel: [T3 {"seconds since 1Jan1904"=timestamp(0 s since 1904-01-01), "Data"=""} ("ActionDataCluster") T3 {"seconds since 1Jan1904"=timestamp(0 s since 1904-01-01), "Data"=""} ("ActionDataCluster") w257 T3 {"seconds since 1Jan1904"=timestamp(0 s since 1904-01-01), "Data"=""} ("ActionDataCluster")] -> w241
      tunnel: w240 -> [_ _ _ w269]
      frame "Wait Send Queue Ready", Default {
        n215 = global read "CommonClientNetworkInterfaceGlobalVariables.vi" "Send Data Queue"() -> (w246:refnum<queue>)
        n216 = Get Queue Status(queue=w246) -> (error out=w250:errorcluster)  [unwired: 2 in, 7 out]
        n217 = Select(t=T4."Wait Send Queue Ready", s=w250, f=T4."Wait Receive Queue Ready") -> (s? t:f=w249:T4)
      }
      frame "Wait Receive Queue Ready" {
        n218 = global read "CommonClientNetworkInterfaceGlobalVariables.vi" "Receive Data Queue"() -> (w252:refnum<queue>)
        n219 = Get Queue Status(queue=w252) -> (error out=w256:errorcluster)  [unwired: 2 in, 7 out]
        n220 = Select(t=T4."Wait Receive Queue Ready", s=w256, f=T4."Poll Read Queue") -> (s? t:f=w253:T4)
      }
      frame "Poll Read Queue" {
        n221 = Obtain Queue(name (unnamed)="FIELD_STATUS", element data type=T3 {"seconds since 1Jan1904"=timestamp(0 s since 1904-01-01), "Data"=""} ("ActionDataCluster")) -> (queue out=w261:refnum<queue>, error out=w259:errorcluster)  [unwired: 3 in, 1 out]
        n222 = Dequeue Element(queue=w261, error in (no error)=w259) -> (element=w257:T3)  [unwired: 1 in, 3 out]
      }
      frame "Process Data" {
        # "TODO: add timestamp reordering"
        n223 = Unbundle By Name(w269) -> ("Data"=w271:string)  [unwired: 1 out]
        n224 = Unflatten From String(type=T6 {"Round"=0, "FieldArray"=[]} ("FieldDataCluster"), binary string=w271) -> (value=w268:T6)  [unwired: 3 in, 2 out]
        n225 = Unbundle By Name(w268) -> ("Round"=w263:u32, "FieldArray"=w265:T7)
        n226 = call "FieldRenderer.vi"("FieldArray"=w265) -> ("Field Picture"=→"Game Field":picture)
        n227 = Number To Decimal String(number=w263) -> (decimal integer string=→"Turns":string)  [unwired: 1 in]
      }
    }
  }
  n228 = while {
    shift-right: [w276] -> _
    shift-left: T4."Wait Send Queue Ready" -> [w273]
    shift-right: [w274] -> _
    shift-left: T3 {"seconds since 1Jan1904"=timestamp(0 s since 1904-01-01), "Data"=""} ("ActionDataCluster") -> [w275]
    stop <- FALSE stop-if-true
    # "Option Update Handler"
    n229 = case shown="\"Wait Send Queue Ready\", Default" w273 {
      tunnel: [w282 w286 T4."Process Data" T4."Poll Read Queue"] -> w276
      tunnel: [T3 {"seconds since 1Jan1904"=timestamp(0 s since 1904-01-01), "Data"=""} ("ActionDataCluster") T3 {"seconds since 1Jan1904"=timestamp(0 s since 1904-01-01), "Data"=""} ("ActionDataCluster") w291 T3 {"seconds since 1Jan1904"=timestamp(0 s since 1904-01-01), "Data"=""} ("ActionDataCluster")] -> w274
      tunnel: w275 -> [_ _ _ w314]
      frame "Wait Send Queue Ready", Default {
        n230 = global read "CommonClientNetworkInterfaceGlobalVariables.vi" "Send Data Queue"() -> (w279:refnum<queue>)
        n231 = Get Queue Status(queue=w279) -> (error out=w283:errorcluster)  [unwired: 2 in, 7 out]
        n232 = Select(t=T4."Wait Send Queue Ready", s=w283, f=T4."Wait Receive Queue Ready") -> (s? t:f=w282:T4)
      }
      frame "Wait Receive Queue Ready" {
        n233 = global read "CommonClientNetworkInterfaceGlobalVariables.vi" "Receive Data Queue"() -> (w285:refnum<queue>)
        n234 = Get Queue Status(queue=w285) -> (error out=w289:errorcluster)  [unwired: 2 in, 7 out]
        n235 = Select(t=T4."Wait Receive Queue Ready", s=w289, f=T4."Poll Read Queue") -> (s? t:f=w286:T4)
      }
      frame "Poll Read Queue" {
        n236 = Obtain Queue(name (unnamed)="OPTION_UPDATE", element data type=T3 {"seconds since 1Jan1904"=timestamp(0 s since 1904-01-01), "Data"=""} ("ActionDataCluster")) -> (queue out=w294:refnum<queue>, error out=w292:errorcluster)  [unwired: 3 in, 1 out]
        n237 = Dequeue Element(queue=w294, error in (no error)=w292) -> (element=w291:T3)  [unwired: 1 in, 3 out]
      }
      frame "Process Data" {
        n238 = Unbundle By Name(w314) -> ("Data"=w313:string)  [unwired: 1 out]
        n239 = Unflatten From String(type=map{string, u32} {} ("Options"), binary string=w313) -> (value=w306:map{string, u32})  [unwired: 3 in, 2 out]
        n240 = Look In Map(map=w306, key="city_density", default value=u32 10) -> (value=w298:u32)  [unwired: 1 out]
        n241 = Look In Map(map=w306, key="mountain_density", default value=u32 10) -> (value=w297:u32)  [unwired: 1 out]
        n242 = Look In Map(map=w306, key="width", default value=u32 10) -> (value=w299:u32)  [unwired: 1 out]
        n243 = Look In Map(map=w306, key="speed", default value=u32 1) -> (value=w296:u32)  [unwired: 1 out]
        n244 = Look In Map(map=w306, key="height", default value=u32 10) -> (value=w300:u32)  [unwired: 1 out]
        n245 = global write "ClientGlobalVariables.vi" "width"(w299) -> ()
        n246 = global write "ClientGlobalVariables.vi" "city_density"(w298) -> ()
        n247 = global write "ClientGlobalVariables.vi" "mountain_density"(w297) -> ()
        n248 = global write "ClientGlobalVariables.vi" "speed"(w296) -> ()
        n249 = global write "ClientGlobalVariables.vi" "height"(w300) -> ()
      }
    }
  }
  n250 = while {
    shift-right: [w320] -> _
    shift-left: T4."Wait Send Queue Ready" -> [w317]
    shift-right: [w318] -> _
    shift-left: T3 {"seconds since 1Jan1904"=timestamp(0 s since 1904-01-01), "Data"=""} ("ActionDataCluster") -> [w319]
    stop <- FALSE stop-if-true
    # "Player Update Handler"
    n251 = case shown="\"Wait Send Queue Ready\", Default" w317 {
      tunnel: [w326 w330 T4."Process Data" T4."Poll Read Queue"] -> w320
      tunnel: [T3 {"seconds since 1Jan1904"=timestamp(0 s since 1904-01-01), "Data"=""} ("ActionDataCluster") T3 {"seconds since 1Jan1904"=timestamp(0 s since 1904-01-01), "Data"=""} ("ActionDataCluster") w335 T3 {"seconds since 1Jan1904"=timestamp(0 s since 1904-01-01), "Data"=""} ("ActionDataCluster")] -> w318
      tunnel: w319 -> [_ _ _ w347]
      frame "Wait Send Queue Ready", Default {
        n252 = global read "CommonClientNetworkInterfaceGlobalVariables.vi" "Send Data Queue"() -> (w323:refnum<queue>)
        n253 = Get Queue Status(queue=w323) -> (error out=w327:errorcluster)  [unwired: 2 in, 7 out]
        n254 = Select(t=T4."Wait Send Queue Ready", s=w327, f=T4."Wait Receive Queue Ready") -> (s? t:f=w326:T4)
      }
      frame "Wait Receive Queue Ready" {
        n255 = global read "CommonClientNetworkInterfaceGlobalVariables.vi" "Receive Data Queue"() -> (w329:refnum<queue>)
        n256 = Get Queue Status(queue=w329) -> (error out=w333:errorcluster)  [unwired: 2 in, 7 out]
        n257 = Select(t=T4."Wait Receive Queue Ready", s=w333, f=T4."Poll Read Queue") -> (s? t:f=w330:T4)
      }
      frame "Poll Read Queue" {
        n258 = Obtain Queue(name (unnamed)="PLAYER_UPDATE", element data type=T3 {"seconds since 1Jan1904"=timestamp(0 s since 1904-01-01), "Data"=""} ("ActionDataCluster")) -> (queue out=w338:refnum<queue>, error out=w336:errorcluster)  [unwired: 3 in, 1 out]
        n259 = Dequeue Element(queue=w338, error in (no error)=w336) -> (element=w335:T3)  [unwired: 1 in, 3 out]
      }
      frame "Process Data" {
        n260 = Unbundle By Name(w347) -> ("Data"=w346:string)  [unwired: 1 out]
        n261 = Unflatten From String(type=T8 {} ("PlayerInfoMap"), binary string=w346) -> (value=w342:T8)  [unwired: 3 in, 2 out]
        n262 = global write "ClientGlobalVariables.vi" "PlayerInfoMap"(w342) -> ()
        n263 = for {
          tunnel: w342 -> [w374] mode=indexing
          shift-right: [w372] -> w343
          shift-left: string[][] [] -> [w373]
          shift-right: [w359] -> w340
          shift-left: T2 [] ("Array 2") -> [w358]
          (unwired) u32 0 ("PlayerInfo.Color")
          n264 = Unbundle By Name(w374) -> ("ID"=w362:u32, "PlayerInfo.Name"=w354:string, "PlayerInfo.Team"=w353:u8, "PlayerInfo.Host"=w355:bool, "PlayerInfo.Ready"=w356:bool, "PlayerInfo.Alive"=w369:bool, "PlayerInfo.Color"=w352:u32, "PlayerInfo.Lands"=w360:set{cluster{"Row":u32, "Column":u32}}, "PlayerInfo.Army"=w366:u32)  [unwired: 1 out]
          n265 = Number To Decimal String(number=w362) -> ()  [unwired: 1 in, 1 out]
          n266 = Number To Decimal String(number=w362) -> ()  [unwired: 1 in, 1 out]
          n267 = Number To Decimal String(number=w353) -> ()  [unwired: 1 in, 1 out]
          n268 = Number To Decimal String(number=w353) -> ()  [unwired: 1 in, 1 out]
          n269 = Build Cluster Array(w360) -> (w368:T10)
          n270 = Bundle By Name(cluster=T9 {"Color"=0, "Host"=FALSE, "Name"="", "Team"=0, "Ready"=FALSE} ("Cluster"), "Color"=w352, "Host"=w355, "Name"=w354, "Team"=w353, "Ready"=w356) -> (w350:T9)
          n271 = Array Size(array=w368) -> (size(s)=w367:i32)
          n272 = Insert Into Array(array=w358, new element=w350) -> (w359:T2)  [unwired: 1 in]
          n273 = Select(t="ALIVE", s=w369, f="DEAD...") -> (s? t:f=w365:string)
          n274 = Number To Decimal String(number=w367) -> (decimal integer string=w361:string)  [unwired: 1 in]
          n275 = Number To Decimal String(number=w366) -> (decimal integer string=w364:string)  [unwired: 1 in]
          n276 = Insert Into Array(array=string[] [], new element #1=w354, new element #2=w365, new element #3=w361, new element #4=w364) -> (w363:string[])  [unwired: 1 in]
          n277 = Insert Into Array(array=w373, new element=w363) -> (w372:string[][])  [unwired: 2 in]
        }
        "In-game Player List" <- w343
        "Lobby Player List" <- w340
      }
    }
  }
